vi "Test Non wired error.vi"() -> ()   [LabVIEW 2014, in "Complex Numbers.lvlib"]
uses:
  Complex Numbers.lvlib
  <vilib>/Aledyne-TSXperts/Arduino Compatible Compiler for LabVIEW/Arduino Compatible Compiler for LabVIEW.lvlib
panel:
  out "error out":errorcluster
  in  "error in (no error)":errorcluster
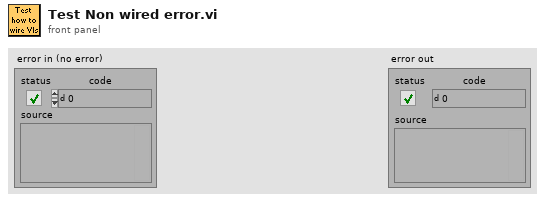
[diagram p1: front panel]
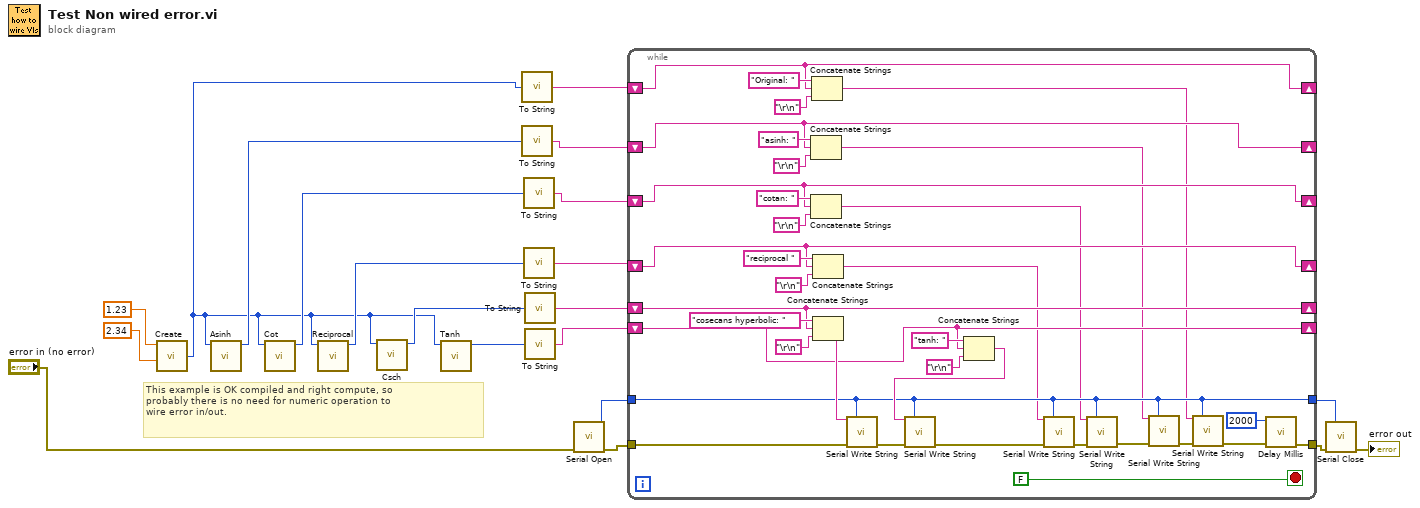
[diagram p0: block diagram]
diagram:
  # "This example is OK compiled and right compute, so\nprobably there is no need for numeric operation to\nwire error in/out."
  n1 = call "Create.vi"("Imag"=2.34, "Real"=1.23) -> ("Complex"=w2:u32)  [unwired: 3 in, 1 out]
  n2 = call "Asinh.vi"("A"=w2) -> ("arcsinh(A)"=w6:u32)  [unwired: 9 in, 1 out]
  n3 = call "Cot.vi"("A"=w2) -> ("cotan(A)"=w7:u32)  [unwired: 9 in, 1 out]
  n4 = call "Reciprocal.vi"("A"=w2) -> ("reciprocal A"=w4:u32)  [unwired: 9 in, 1 out]
  n5 = call "Csch.vi"("A"=w2) -> ("csch(A)"=w5:u32)  [unwired: 9 in, 1 out]
  n6 = call "Tanh.vi"("A"=w2) -> ("tanh(A)"=w3:u32)  [unwired: 9 in, 1 out]
  n7 = call "To String.vi"("Complex number"=w2) -> ("String complex num."=w11:string)
  n8 = call "To String.vi"("Complex number"=w6) -> ("String complex num."=w10:string)
  n9 = call "To String.vi"("Complex number"=w7) -> ("String complex num."=w9:string)
  n10 = call "To String.vi"("Complex number"=w4) -> ("String complex num."=w8:string)
  n11 = call "To String.vi"("Complex number"=w5) -> ("String complex num."=w12:string)
  n12 = call "To String.vi"("Complex number"=w3) -> ("String complex num."=w13:string)
  n13 = call <vilib>:"Serial Open.vi"("error in (no error)"="error in (no error)") -> ("Instance"=w18:u8, "error out"=w20:errorcluster)  [unwired: 13 in]
  n14 = while {
    tunnel: w20 -> [w52]
    tunnel: [w54] -> w19
    tunnel: w18 -> [w29]
    tunnel: [w29] -> w17
    shift-right: [w45] -> _
    shift-left: w12 -> [w45]
    shift-right: [w43] -> _
    shift-left: w13 -> [w43]
    shift-right: [w25] -> _
    shift-left: w8 -> [w25]
    shift-right: [w26] -> _
    shift-left: w9 -> [w26]
    shift-right: [w27] -> _
    shift-left: w10 -> [w27]
    shift-right: [w28] -> _
    shift-left: w11 -> [w28]
    stop <- FALSE stop-if-true
    n15 = Concatenate Strings("asinh: " ("string"), w27, "\r\n") -> (w22:string)
    n16 = Concatenate Strings("cotan: " ("string"), w26, "\r\n") -> (w23:string)
    n17 = Concatenate Strings("Original: " ("string"), w28, "\r\n") -> (w21:string)
    n18 = Concatenate Strings("reciprocal " ("string"), w25, "\r\n") -> (w24:string)
    n19 = Concatenate Strings("cosecans hyperbolic: " ("string"), w45, "\r\n") -> (w48:string)
    n20 = call <vilib>:"Serial Write String.vi"("String"=w48, "Instance"=w29, "error in (no error)"=w52) -> ("error out"=w51:errorcluster)  [unwired: 12 in]
    n21 = Concatenate Strings("tanh: " ("string"), w43, "\r\n") -> (w47:string)
    n22 = call <vilib>:"Serial Write String.vi"("String"=w47, "Instance"=w29, "error in (no error)"=w51) -> ("error out"=w31:errorcluster)  [unwired: 12 in]
    n23 = call <vilib>:"Serial Write String.vi"("String"=w24, "Instance"=w29, "error in (no error)"=w31) -> ("error out"=w32:errorcluster)  [unwired: 12 in]
    n24 = call <vilib>:"Serial Write String.vi"("String"=w23, "Instance"=w29, "error in (no error)"=w32) -> ("error out"=w33:errorcluster)  [unwired: 12 in]
    n25 = call <vilib>:"Serial Write String.vi"("String"=w22, "Instance"=w29, "error in (no error)"=w33) -> ("error out"=w34:errorcluster)  [unwired: 12 in]
    n26 = call <vilib>:"Serial Write String.vi"("String"=w21, "Instance"=w29, "error in (no error)"=w34) -> ("error out"=w30:errorcluster)  [unwired: 12 in]
    n27 = call <vilib>:"Delay Millis.vi"("error in (no error)"=w30, "delay"=u32 2000) -> ("error out"=w54:errorcluster)  [unwired: 9 in]
  }
  n28 = call <vilib>:"Serial Close.vi"("Instance"=w17, "error in (no error)"=w19) -> ("error out"=→"error out":errorcluster)  [unwired: 13 in]
